vi "DSF.Engine.Memory.ObjectPool.Bundle.Valid.vi"(8 "error in (no error)":errorcluster, 11 "ObjectPool Bundle in":refnum<class "DSF.Engine.Memory.ObjectPool.Bundle.lvclass">) -> (0 "error out":errorcluster, 2 "valid?":bool, 3 "ObjectPool Bundle out":refnum<class "DSF.Engine.Memory.ObjectPool.Bundle.lvclass">)   [LabVIEW 2016, in "DSF.Engine.lvlib" / "DSF.Engine.Memory.ObjectPool.Bundle.lvclass"]
uses:
  DSF.Engine.Memory.ObjectPool.Bundle.lvclass
  DSF.Engine.Memory.ObjectPool.Bundle.lvclass/DSF.Engine.Memory.ObjectPool.Bundle.ctl
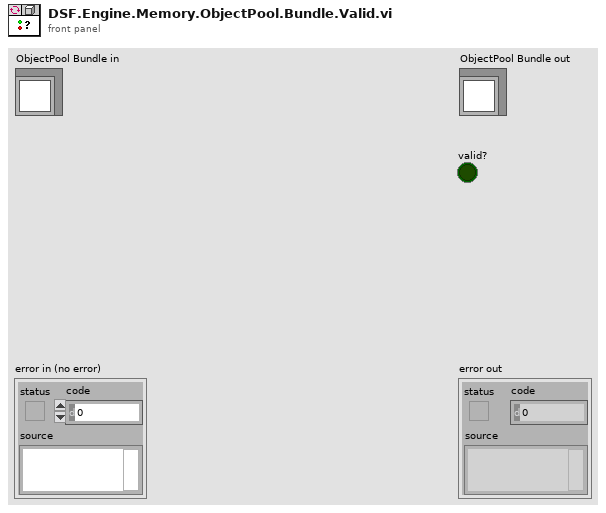
[diagram p1: front panel]
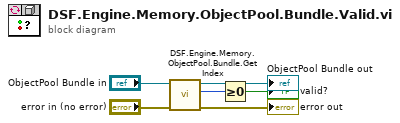
[diagram p0: block diagram]
diagram:
  n1 = call "DSF.Engine.Memory.ObjectPool.Bundle.Get Index.vi"("error in (no error)"="error in (no error)", "ObjectPool Bundle in"="ObjectPool Bundle in") -> ("error out"=→"error out":errorcluster, "Index"=w4:i32, "ObjectPool Bundle out"=→"ObjectPool Bundle out":refnum<class "DSF.Engine.Memory.ObjectPool.Bundle.lvclass">)  [unwired: 7 in]
  n2 = Greater Or Equal To 0?(x=w4) -> (x >= 0?=→"valid?":bool)
